vi "Complex Trigger And-Or condition.vi"(8 "error in (no error)":errorcluster, 10 "Complex trigger compare OR or AND":u16(ring) items=["OR", "AND"], 11 "VISA resource name":refnum<visa-resource-name>) -> (0 "error out":errorcluster, 3 "VISA resource name out":refnum<visa-resource-name>)   [LabVIEW 2017, in "Sefram DAS220.lvlib"]
doc: "Defines the relation between each condition in the list.\nFor example : A1 > 0,5V; A2 > 1V.\nIf relation AND selected : trig if 2 conditions are TRUE.\nIf relation OR selected : trig if at least one condition is TRUE."
uses:
  <instrlib>/Sefram DAS220/Sefram DAS220.lvlib
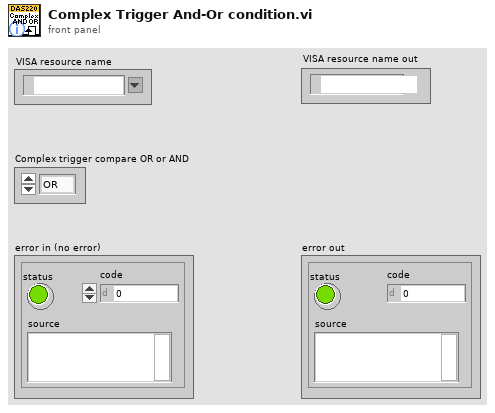
[diagram p1: front panel]
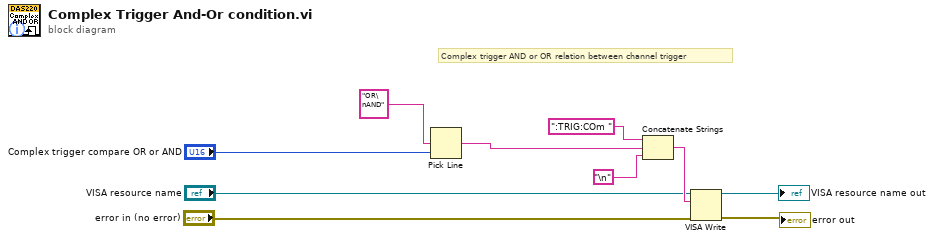
[diagram p0: block diagram]
diagram:
  # "Complex trigger AND or OR relation between channel trigger"
  n1 = Pick Line(multi-line string="OR\nAND", line index="Complex trigger compare OR or AND") -> (output string=w3:string)  [unwired: 1 in]
  n2 = Concatenate Strings(":TRIG:COm " ("string"), w3, "\n") -> (w10:string)
  n3 = VISA Write(VISA resource name="VISA resource name", write buffer=w10, error in (no error)="error in (no error)") -> (VISA resource name out=→"VISA resource name out":refnum<visa-resource-name>, error out=→"error out":errorcluster)  [unwired: 1 out]
